vi "PH_Cam_BaseClass.Setting Unpacker.vi"(2 "Cam Settings Array":string[](array[string]), 5 "error in (no error)":errorcluster) -> (16 "Cam Setting Information":string="N/A", 17 "Cam Settings":T1={"Cam ID"="N/A", "Gain"=nan, "Brightness"=nan, "Shutter"=nan, "Mode"=-1}, 19 "error out":errorcluster)   [LabVIEW 2014, in "PH_Cam_BaseClass.lvlib"]
doc: "This VI gets the cam settings from an string, converts them to a string array and gives out the result as customized cluster."
uses:
  PH_Cam_BaseClass.lvlib
  PH_Cam_BaseClass.Settings.ctl
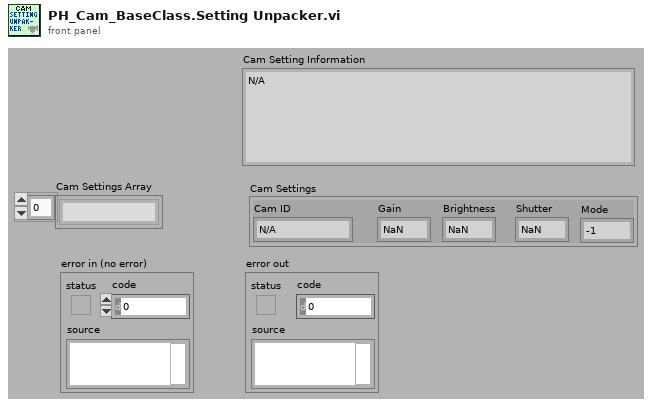
[diagram p1: front panel]
types:
  T1 = typedef "PH_Cam_BaseClass.lvlib/PH_Cam_BaseClass.Settings.ctl" = cluster{"Cam ID":string, "Gain":dbl, "Brightness":dbl, "Shutter":dbl, "Mode":i32}
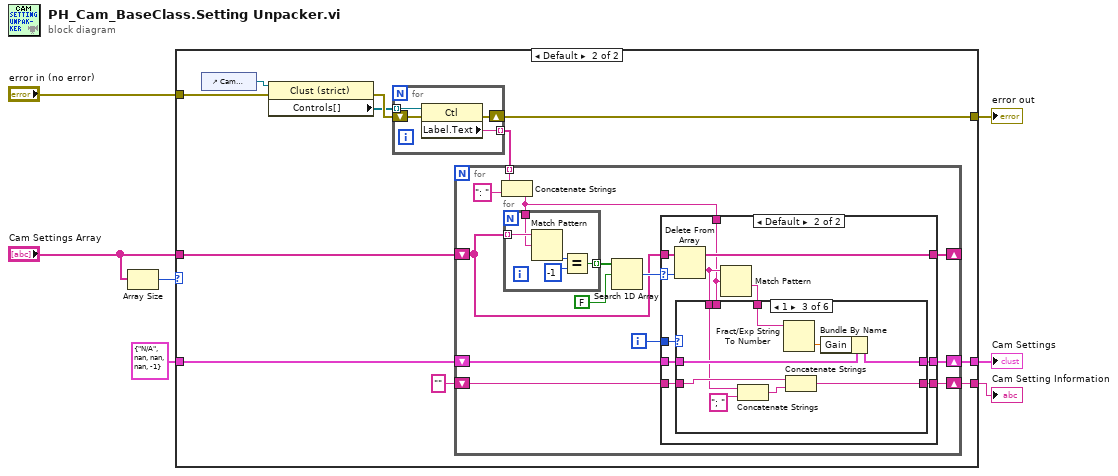
[diagram p0: block diagram]
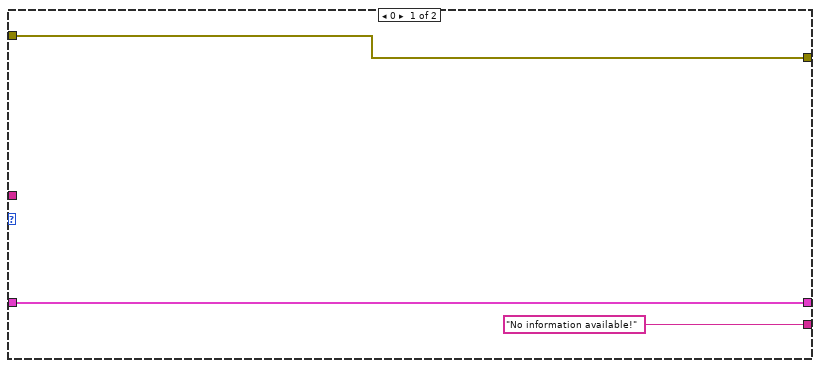
[diagram p2: hidden frame]
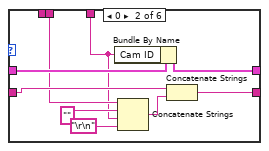
[diagram p5: hidden frame]
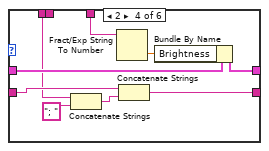
[diagram p6: hidden frame]
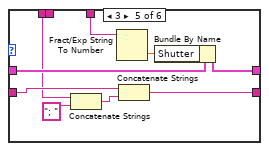
[diagram p7: hidden frame]
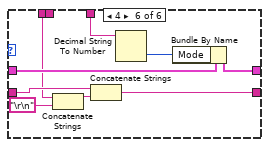
[diagram p8: hidden frame]
diagram:
  n1 = Array Size(array="Cam Settings Array") -> (size(s)=w3:i32)
  n2 = case shown="Default" w3 {
    tunnel: [w10 w21] -> w7
    tunnel: "error in (no error)" -> [w10 w18]
    tunnel: [w8 w17] -> w5
    tunnel: "Cam Settings Array" -> [_ w15]
    tunnel: ["No information available!" w14] -> w2
    tunnel: T1 {"Cam ID"="N/A", "Gain"=nan, "Brightness"=nan, "Shutter"=nan, "Mode"=-1} ("Cam Setting Template") -> [w8 w11]
    frame 0 {
    }
    frame Default {
      n3 = control-ref of="Cam Settings"() -> (w12:refnum<vi>)
      n4 = property class="Clust (strict)"(reference=w12, error in=w18) -> (error out=w20:errorcluster, "Controls[]"=w19:refnum<vi>[])  [unwired: 1 out]
      n5 = for {
        tunnel: w19 -> [w104] mode=indexing
        tunnel: [w103] -> w16 mode=indexing
        shift-right: [w101] -> w21
        shift-left: w20 -> [w102]
        n6 = property class="Ctl"(reference=w104, error in=w102) -> (error out=w101:errorcluster, "Label.Text"=w103:string)  [unwired: 1 out]
      }
      n7 = for {
        tunnel: w16 -> [w34] mode=indexing
        shift-right: [w30] -> _
        shift-left: w15 -> [w25]
        shift-right: [w26] -> w17
        shift-left: w11 -> [w27]
        shift-right: [w23] -> w14
        shift-left: "" -> [w22]
        i -> [w24]
        n8 = Concatenate Strings(w34, ": " ("string")) -> (w28:string)
        n9 = for {
          tunnel: w25 -> [w100] mode=indexing
          tunnel: w28 -> [w99]
          tunnel: [w96] -> w32 mode=indexing
          n10 = Match Pattern(string=w100, regular expression=w99) -> (offset past match=w98:i32)  [unwired: 1 in, 3 out]
          n11 = Equal?(x=w98, y=-1) -> (x = y?=w96:bool)
        }
        n12 = Search 1D Array(1D array=w32, element=FALSE) -> (index of element=w29:i32)  [unwired: 1 in]
        n13 = case shown="Default" w29 {
          selector: w29 -> [_ w46]
          tunnel: [w37 w48] -> w30
          tunnel: w25 -> [w37 w47]
          tunnel: w28 -> [_ w38]
          tunnel: w27 -> [w36 w45]
          tunnel: [w36 w44] -> w26
          tunnel: w24 -> [_ w42]
          tunnel: [w35 w40] -> w23
          tunnel: w22 -> [w35 w39]
          frame -1 {
          }
          frame Default {
            n14 = Delete From Array(array=w47, index=w46) -> (deleted portion=w41:string, array with subset deleted=w48:string[])  [unwired: 1 in]
            n15 = Match Pattern(string=w41, regular expression=w38) -> (after substring=w43:string)  [unwired: 1 in, 3 out]
            n16 = case shown="1" w42 {
              tunnel: w45 -> [w50 w59 w68 w77 w86 w95]
              tunnel: [w50 w58 w67 w76 w85 w94] -> w44
              tunnel: w43 -> [_ w51 w66 w75 w84 w93]
              tunnel: w41 -> [_ _ w61 w70 w79 w88]
              tunnel: [w49 w56 w62 w71 w80 w87] -> w40
              tunnel: w39 -> [w49 w54 w63 w72 w81 w89]
              tunnel: w38 -> [_ w53 _ _ _ _]
              frame Default {
              }
              frame 0 {
                n17 = Bundle By Name(cluster=w59, "Cam ID"=w51) -> (w58:T1)
                n18 = Concatenate Strings(w53, "" ("string"), w51, "\r\n") -> (w55:string)
                n19 = Concatenate Strings(w54, w55) -> (w56:string)
              }
              frame 1 {
                n20 = Concatenate Strings(w61, "; " ("string")) -> (w64:string)
                n21 = Fract/Exp String To Number(string=w66) -> (number=w65:dbl)  [unwired: 3 in, 1 out]
                n22 = Concatenate Strings(w63, w64) -> (w62:string)
                n23 = Bundle By Name(cluster=w68, "Gain"=w65) -> (w67:T1)
              }
              frame 2 {
                n24 = Concatenate Strings(w70, "; " ("string")) -> (w73:string)
                n25 = Fract/Exp String To Number(string=w75) -> (number=w74:dbl)  [unwired: 3 in, 1 out]
                n26 = Concatenate Strings(w72, w73) -> (w71:string)
                n27 = Bundle By Name(cluster=w77, "Brightness"=w74) -> (w76:T1)
              }
              frame 3 {
                n28 = Concatenate Strings(w79, "; " ("string")) -> (w82:string)
                n29 = Fract/Exp String To Number(string=w84) -> (number=w83:dbl)  [unwired: 3 in, 1 out]
                n30 = Concatenate Strings(w81, w82) -> (w80:string)
                n31 = Bundle By Name(cluster=w86, "Shutter"=w83) -> (w85:T1)
              }
              frame 4 {
                n32 = Concatenate Strings(w88, "\r\n") -> (w90:string)
                n33 = Concatenate Strings(w89, w90) -> (w87:string)
                n34 = Decimal String To Number(string=w93) -> (number=w92:i32)  [unwired: 2 in, 1 out]
                n35 = Bundle By Name(cluster=w95, "Mode"=w92) -> (w94:T1)
              }
            }
          }
        }
      }
    }
  }
  "error out" <- w7
  "Cam Settings" <- w5
  "Cam Setting Information" <- w2
